vi "Get Debug.vi"(8 "error in (no error)":errorcluster, 11 "AdbBridge in":refnum<class "Adb Bridge.lvclass">) -> (0 "error out":errorcluster, 2 "dbg msg":string, 3 "AdbBridge out":refnum<class "Adb Bridge.lvclass">)   [LabVIEW 2016, in "Adb Bridge.lvclass"]
uses:
  Adb Bridge.lvclass
  Adb Bridge.lvclass/Adb Bridge.ctl
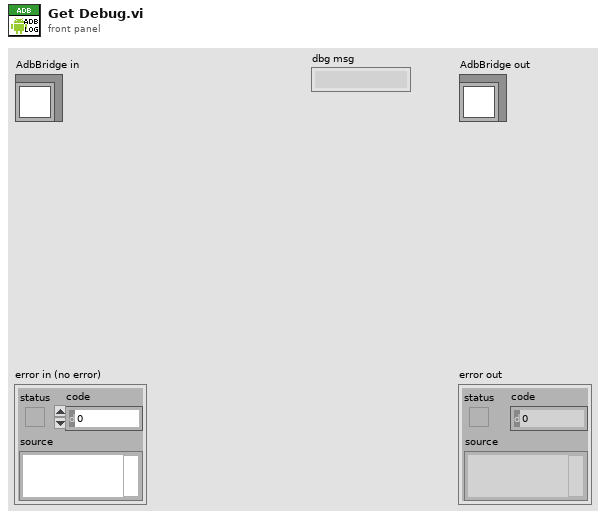
[diagram p1: front panel]
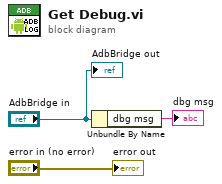
[diagram p0: block diagram]
diagram:
  n1 = Unbundle By Name("AdbBridge in") -> ("dbg msg"=→"dbg msg":string)
  "error out" <- "error in (no error)"
  "AdbBridge out" <- "AdbBridge in"
